vi "Get Server Internal UEs.vi"(11 "OOP Server in":refnum<class "helloWServer.lvclass">) -> (2 "Server Internal UEs":T1, 3 "OOP Server out":refnum<class "helloWServer.lvclass">)   [LabVIEW 2020, in "helloWServer.lvlib" / "helloWServer.lvclass"]
uses:
  helloWServer.lvclass
  typeDefs/Server Internal UEs.ctl
  helloWServer.lvclass/helloWServer.ctl
  typeDefs/Server Internal Message.ctl
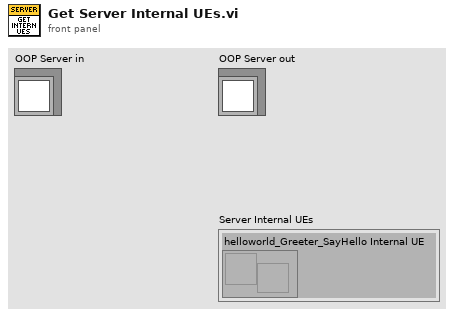
[diagram p1: front panel]
types:
  T1 = typedef "helloWServer.lvlib/helloWServer.lvclass/Server Internal UEs.ctl" = cluster{"helloworld_Greeter_SayHello Internal UE":refnum<user-event>}
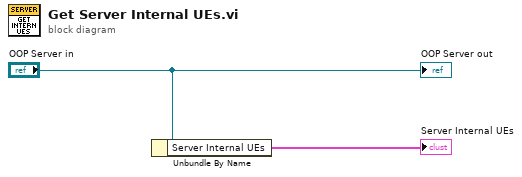
[diagram p0: block diagram]
diagram:
  n1 = Unbundle By Name("OOP Server in") -> ("Server Internal UEs"=→"Server Internal UEs":T1)
  "OOP Server out" <- "OOP Server in"
